vi "Read_AI_Module.vi"(8 "error in (no error)":errorcluster, 11 "USB-87Pn in":refnum<class "USB-87Pn.lvclass">) -> (0 "error out":errorcluster, 2 "AI float":sgl[][](array[numeric]), 3 "USB-87Pn out":refnum<class "USB-87Pn.lvclass">)   [LabVIEW 2019, in "USB-87Pn.lvlib" / "USB-87Pn.lvclass"]
uses:
  USB-87Pn.lvclass
  USB-87Pn.lvclass/USB-87Pn.ctl
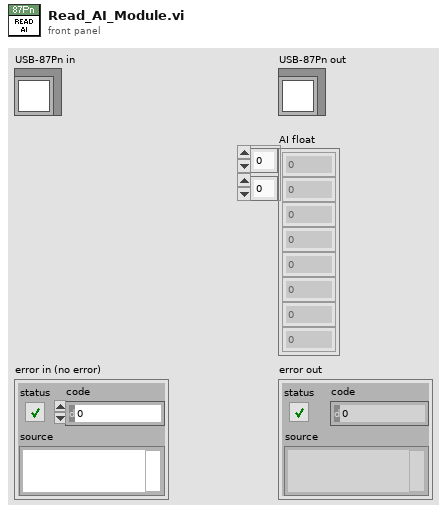
[diagram p1: front panel]
types:
  T1 = typedef "USB-87Pn.lvlib/USB-87Pn.lvclass/AI_Module_Data.ctl" = cluster{"Module_Data":T2, "AI_Channels":cluster{"Enabled":bool, "Alias":string}[]}
  T2 = typedef "USB-87Pn.lvlib/USB-87Pn.lvclass/Module_Data.ctl" = cluster{"Number of Channels":u8, "Address":i16, "Alias":string}
  T3 = cluster{"ComPort":u8, "Address":i16, "Slot":i16, "CheckSum":i16, "TimeOut":i16}
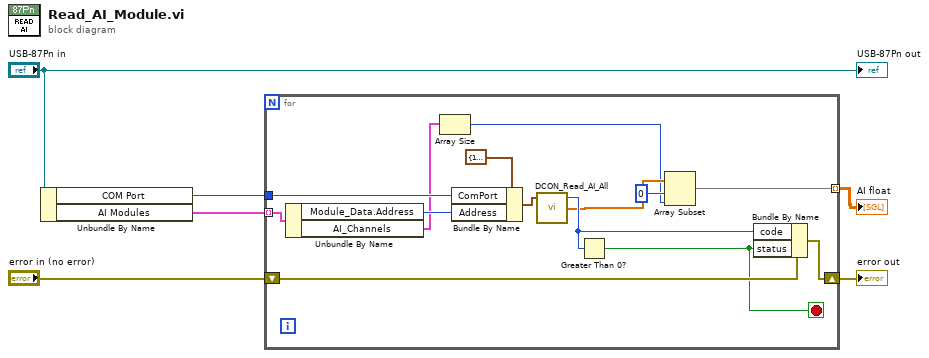
[diagram p0: block diagram]
diagram:
  n1 = Unbundle By Name("USB-87Pn in") -> ("COM Port"=w4:u8, "AI Modules"=w5:T1[])
  n2 = for {
    tunnel: w5 -> [w20] mode=indexing
    tunnel: w4 -> [w18]
    shift-right: [w13] -> w2
    shift-left: "error in (no error)" -> [w15]
    tunnel: [w8] -> w1 mode=indexing
    stop <- w14 stop-if-true
    n3 = Unbundle By Name(w20) -> ("Module_Data.Address"=w19:i16, "AI_Channels"=w11:cluster{"Enabled":bool, "Alias":string}[])
    n4 = Array Size(array=w11) -> (size(s)=w7:i32)
    n5 = Bundle By Name(cluster=T3 {"ComPort"=1, "Address"=0, "Slot"=-1, "CheckSum"=0, "TimeOut"=1000} ("DCON_Module"), "ComPort"=w18, "Address"=w19) -> (w16:T3)
    n6 = call <vilib>:"DCON_Read_AI_All.vi"("DCON_Module"=w16) -> ("AI float"=w10:sgl[], "return"=w12:i16)  [unwired: 2 in, 1 out]
    n7 = Greater Than 0?(x=w12) -> (x > 0?=w14:bool)
    n8 = Array Subset(array=w10, index=0, length=w7) -> (w8:sgl[])
    n9 = Bundle By Name(cluster=w15, "code"=w12, "status"=w14) -> (w13:errorcluster)
  }
  "error out" <- w2
  "AI float" <- w1
  "USB-87Pn out" <- "USB-87Pn in"
